vi "fixPoiPaths.vi"(10 "ItemNames":string[][](array[string]), 11 "loopData":T1) -> (2 "ok":bool, 3 "newPaths":path[](array[path]))   [LabVIEW 2014]
uses:
  typeDefs/loopDataType.ctl
  typeDefs/editControl.ctl
  typeDefs/variantFlat.ctl
  typeDefs/pictChooser.ctl
  <userlib>/_OpenG.lib/file/file.llb/File Exists - Scalar__ogtk.vi
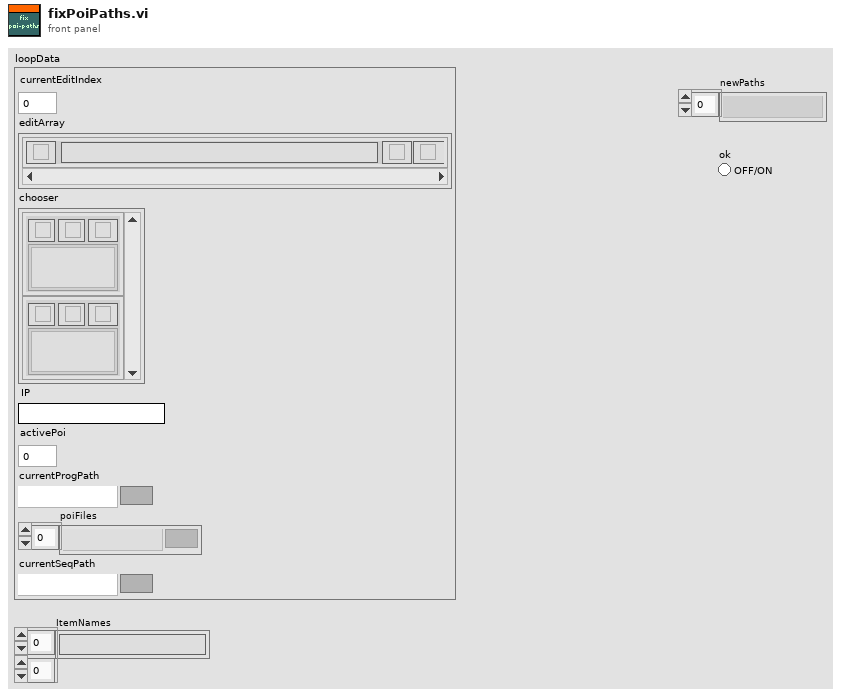
[diagram p1: front panel]
types:
  T1 = typedef "loopDataType.ctl" = cluster{"currentEditIndex":i32, "editArray":T2[], "chooser":T4[], "IP":string, "activePoi":i32, "currentProgPath":path, "poiFiles":path[], "currentSeqPath":path}
  T2 = typedef "editControl.ctl" = cluster{"edit":bool, "info":string, "variantFlat":T3, "codeCluster":cluster{"code":u8[][]}, "del":bool, "ins":bool}
  T3 = typedef "variantFlat.ctl" = cluster{"type string":i16[], "data string":string}
  T4 = typedef "pictChooser.ctl" = cluster{"2D Picture":picture, "load":bool, "Path":path, "Bitmap":u32[][], "del":bool, "paint":bool}
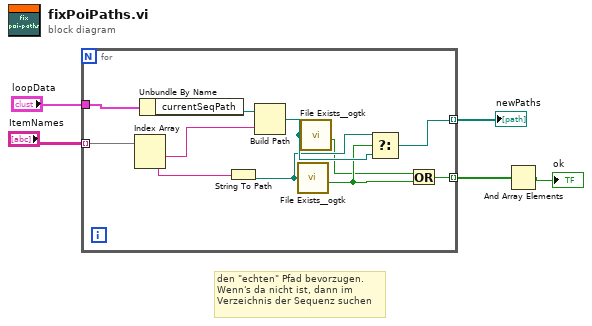
[diagram p0: block diagram]
diagram:
  # "den \"echten\" Pfad bevorzugen.\nWenn's da nicht ist, dann im\nVerzeichnis der Sequenz suchen"
  n1 = for {
    tunnel: [w16] -> w2 mode=indexing
    tunnel: [w11] -> w5 mode=indexing
    tunnel: "loopData" -> [w8]
    tunnel: "ItemNames" -> [w6] mode=indexing
    n2 = Index Array(array=w6) -> (element #1=w9:string, element #2=w12:string)  [unwired: 2 in]
    n3 = Unbundle By Name(w8) -> ("currentSeqPath"=w7:path)
    n4 = String To Path(string=w12) -> (path=w14:path)
    n5 = Build Path(base path=w7, name or relative path=w9) -> (appended path=w15:path)
    n6 = call-poly <userlib>:"File Exists__ogtk.vi"("file path"=w14) -> ("exists"=w13:bool)  [unwired: 6 in, 1 out]
    n7 = call-poly <userlib>:"File Exists__ogtk.vi"("file path"=w15) -> ("exists"=w10:bool)  [unwired: 6 in, 1 out]
    n8 = Select(t=w14, s=w13, f=w15) -> (s? t:f=w16:path)
    n9 = Or(x=w10, y=w13) -> (x .or. y?=w11:bool)
  }
  "newPaths" <- w2
  n10 = And Array Elements(Boolean array=w5) -> (logical AND=→"ok":bool)
